vi "Parse Message Buffer.vi"(7 "flush buffer":bool, 8 "error in":errorcluster, 11 "string in":string) -> (0 "error out":errorcluster, 1 "valid":bool, 3 "message":cluster{"command":u8, "payload":string})   [LabVIEW 2018, in "LIA Host Interface RT.lvclass"]
uses:
  LIA Host Interface RT.lvclass
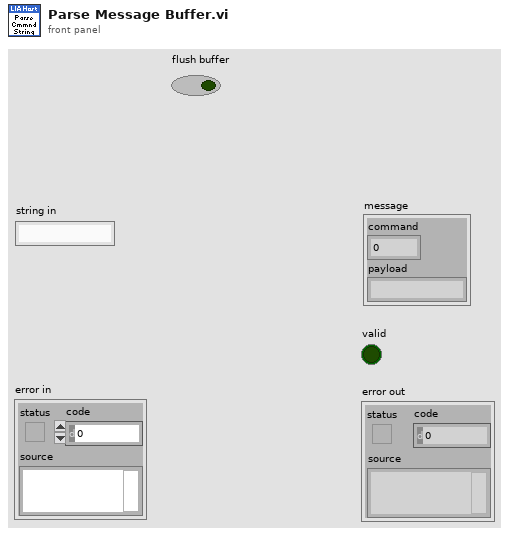
[diagram p1: front panel]
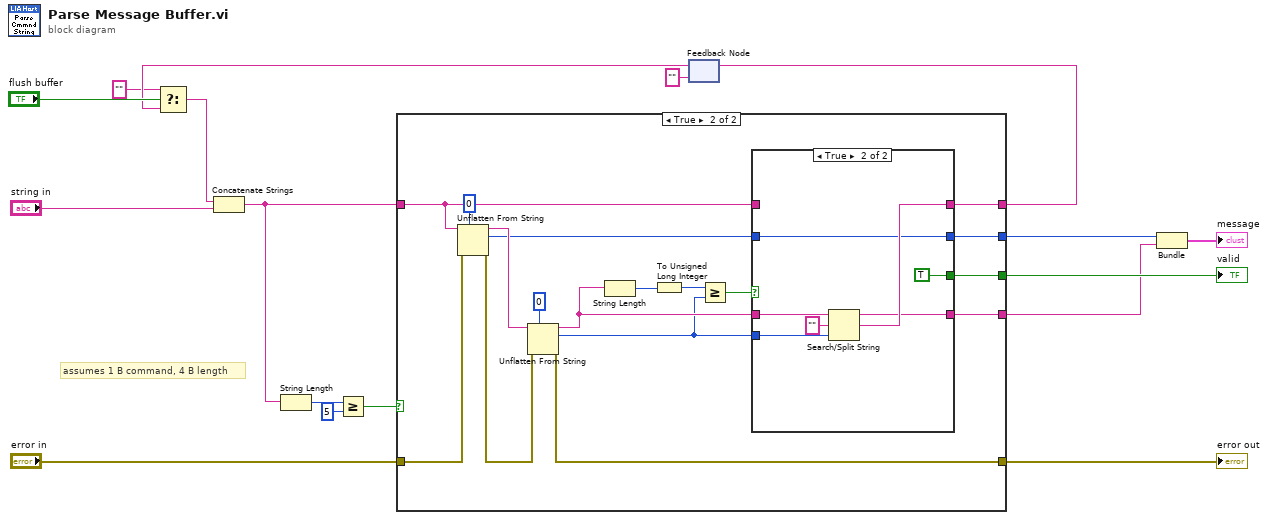
[diagram p0: block diagram]
diagram:
  # "assumes 1 B command, 4 B length"
  n1 = feedback #1("") -> (w3:string)
  n2 = Select(t="", s="flush buffer", f=w3) -> (s? t:f=w1:string)
  n3 = Concatenate Strings(w1, "string in") -> (w12:string)
  n4 = String Length(string=w12) -> (length=w14:i32)
  n5 = Greater Or Equal?(x=w14, y=5) -> (x >= y?=w16:bool)
  n6 = case shown="True" w16 {
    tunnel: w12 -> [w19 w30]
    tunnel: [_ w29] -> w13
    tunnel: "error in" -> [w18 w28]
    tunnel: [w18 w26] -> w10
    tunnel: [w19 w23] -> w5
    tunnel: [_ w22] -> w8
    tunnel: [_ w20] -> w9
    frame False {
    }
    frame True {
      n7 = Unflatten From String(type=u8 0 ("offset (0)"), binary string=w30, error in (no error)=w28) -> (rest of the binary string=w35:string, value=w21:u8, error out=w27:errorcluster)  [unwired: 2 in]
      n8 = Unflatten From String(type=u32 0 ("offset (0)"), binary string=w35, error in (no error)=w27) -> (rest of the binary string=w25:string, value=w24:u32, error out=w26:errorcluster)  [unwired: 2 in]
      n9 = String Length(string=w25) -> (length=w33:i32)
      n10 = To Unsigned Long Integer(number=w33) -> (unsigned 32bit integer=w32:u32)
      n11 = Greater Or Equal?(x=w32, y=w24) -> (x >= y?=w31:bool)
      n12 = case shown="True" w31 {
        tunnel: w30 -> [w37 _]
        tunnel: [w37 w41] -> w23
        tunnel: [_ TRUE] -> w29
        tunnel: w25 -> [_ w44]
        tunnel: w24 -> [_ w43]
        tunnel: [_ w40] -> w22
        tunnel: w21 -> [_ w38]
        tunnel: [_ w38] -> w20
        frame False {
        }
        frame True {
          n13 = Search/Split String(string=w44, search string/char (-)="", offset (0)=w43) -> (substring before match=w40:string, match + rest of string=w41:string)  [unwired: 1 out]
        }
      }
    }
  }
  "error out" <- w10
  "valid" <- w13
  n14 = feedback-in #1(w5) -> ()
  n15 = Bundle("offset (0)"=w9, w8) -> (→"message":cluster{"offset (0)":u8, string})  [unwired: 1 in]
